vi "Register Assert.vi"(4 "Unique ID":string, 6 "Call Chain":string[](array[string]), 7 "Execution time (s)":dbl=-1.0, 8 "error in (no error)":errorcluster, 9 "Succeeded":bool, 10 "Message":string, 11 "Test Manager in":refnum<class "Basic Test Manager.lvclass">) -> (0 "error out":errorcluster, 3 "Test Manager out":refnum<class "Basic Test Manager.lvclass">)   [LabVIEW 2013, in "Caraya.lvlib" / "Basic Test Manager.lvclass"]
uses:
  Basic Test Manager.lvclass
  Test Result/Assert Event Data.ctl
  Test Result/Test Event Data.ctl
  Basic Test Manager.lvclass/Basic Test Manager.ctl
  Test Result/Test Result.lvclass
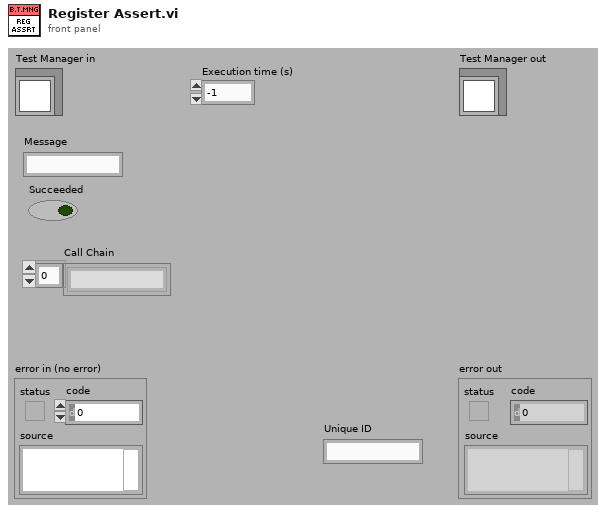
[diagram p1: front panel]
types:
  T1 = typedef "Caraya.lvlib/Test Result.lvclass/Test Event Data.ctl" = cluster{"Label":string, "Argument":variant}
  T2 = typedef "Caraya.lvlib/Test Result.lvclass/Assert Event Data.ctl" = cluster{"Name":string, "Passed":bool, "Call Chain":string[], "Test Error":errorcluster, "Time Stamp":timestamp, "Unique Assert ID":string, "Test Key":string, "Execution time (s)":dbl, "Verbose Explanation":string}
  T3 = typedef "Caraya.lvlib/Test Result.lvclass/Test Event.ctl" = refnum<user-event>
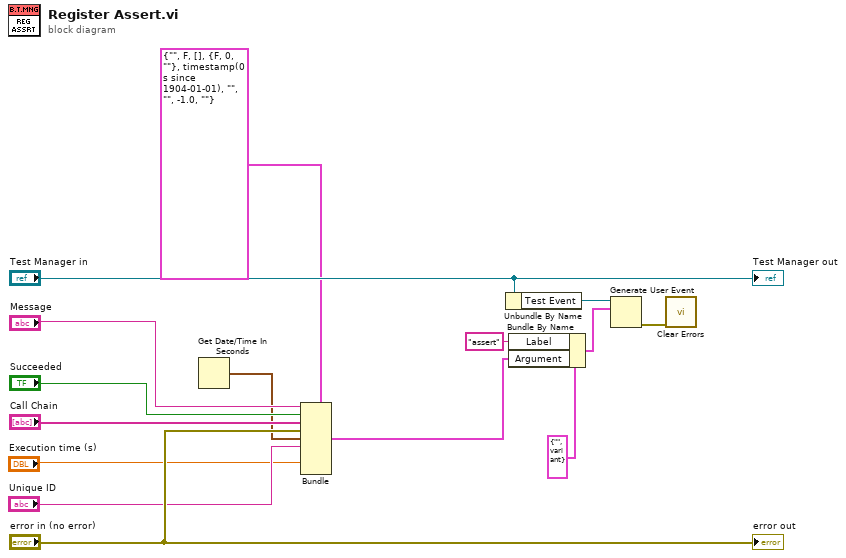
[diagram p0: block diagram]
diagram:
  n1 = Get Date/Time In Seconds() -> (seconds since 1Jan1904=w4:timestamp)
  n2 = Bundle(cluster=T2 {"Name"="", "Passed"=FALSE, "Call Chain"=[], "Test Error"={"status"=FALSE, "code"=0, "source"=""}, "Time Stamp"=timestamp(0 s since 1904-01-01), "Unique Assert ID"="", "Test Key"="", "Execution time (s)"=-1.0, "Verbose Explanation"=""} ("Test Event"), "Name"="Message", "Passed"="Succeeded", "Call Chain"="Call Chain", "Test Error"="error in (no error)", "Time Stamp"=w4, "Unique Assert ID"="Unique ID", "Execution time (s)"="Execution time (s)") -> (w8:T2)  [unwired: 2 in]
  n3 = Unbundle By Name("Test Manager in") -> ("Test Event"=w11:T3)
  n4 = Bundle By Name(cluster=T1 {"Label"="", "Argument"=variant} ("Test Event"), "Label"="assert" ("Message"), "Argument"=w8) -> (w10:T1)
  n5 = Generate User Event(user event=w11, event data cluster=w10) -> (error out=w6:errorcluster)  [unwired: 2 in, 1 out]
  n6 = call <vilib>:"Clear Errors.vi"("error in (no error)"=w6) -> ()  [unwired: 6 in, 1 out]
  "error out" <- "error in (no error)"
  "Test Manager out" <- "Test Manager in"
